vi "Esercitazione 5 - Esercizio per casa, Max Array.vi"() -> ()   [LabVIEW 2018]
panel:
  out "Massimo":dbl
  in  "Array":dbl[](array[numeric])
  # "trovare nell'array il valore massimo"
  # "senza usare il blocco max&min"
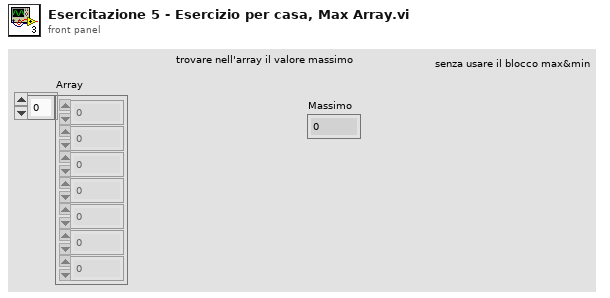
[diagram p1: front panel]
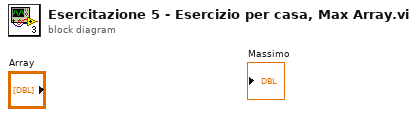
[diagram p0: block diagram]
diagram:
